vi "OAT Verify Resampled Signal (Single Channel).vi"(8 "error in (no error)":errorcluster, 11 "resampled signal":cluster{"r0":dbl, "dr":dbl, "Y":dbl[]} {"r0" format="%.2p"; "dr" format="%.2p"; "Y" format="%.2f"}) -> (0 "error out":errorcluster, 2 "empty signal?":bool, 3 "resampled signal dup":cluster{"r0":dbl, "dr":dbl, "Y":dbl[]} {"r0" format="%.2p"; "dr" format="%.2p"; "Y" format="%.2f"})   [LabVIEW 2017, in "SoundVib_Resampling.lvlib"]
uses:
  <vilib>/addons/Sound and Vibration/Order Analysis/Resample Order Tracking/SoundVib_Resampling.lvlib
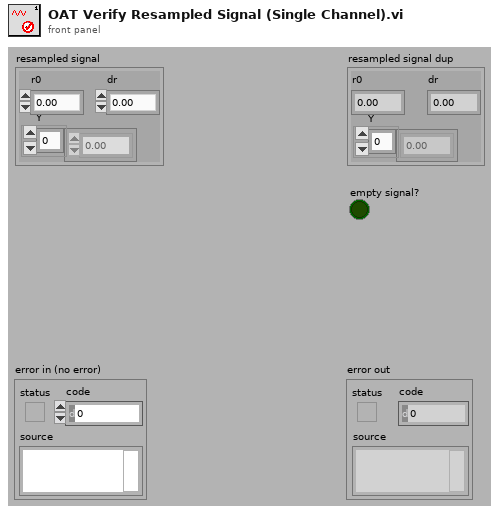
[diagram p1: front panel]
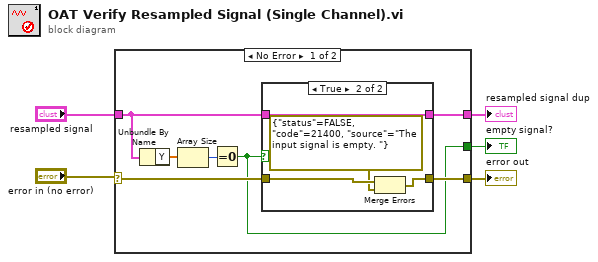
[diagram p0: block diagram]
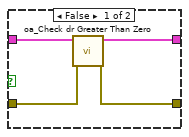
[diagram p2: hidden frame]
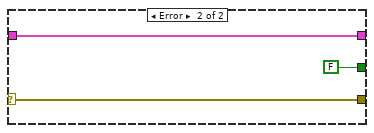
[diagram p3: hidden frame]
diagram:
  n1 = case shown="No Error" "error in (no error)" {
    selector: "error in (no error)" -> [w8 w23]
    tunnel: [w7 w23] -> w4
    tunnel: "resampled signal" -> [w10 w22]
    tunnel: [w9 w22] -> w2
    tunnel: [w6 FALSE] -> w1
    frame No Error {
      n2 = Unbundle By Name(w10) -> ("Y"=w12:dbl[])
      n3 = Array Size(array=w12) -> (size(s)=w11:i32)
      n4 = Equal To 0?(x=w11) -> (x = 0?=w6:bool)
      n5 = case shown="True" w6 {
        tunnel: w10 -> [w16 w20]
        tunnel: [w15 w20] -> w9
        tunnel: w8 -> [w14 w18]
        tunnel: [w13 w19] -> w7
        frame False {
          n6 = call <vilib>:"oa_Check dr Greater Than Zero.vi"("error in (no error)"=w14, "resampled signal"=w16) -> ("error out"=w13:errorcluster, "resampled signal dup"=w15:cluster{"r0":dbl, "dr":dbl, "Y":dbl[]})  [unwired: 8 in]
        }
        frame True {
          n7 = Merge Errors(w18, errorcluster {"status"=FALSE, "code"=21400, "source"="The input signal is empty. "} ("error IO")) -> (w19:errorcluster)
        }
      }
    }
    frame Error {
    }
  }
  "error out" <- w4
  "resampled signal dup" <- w2
  "empty signal?" <- w1
